vi "De-Classify Error Call Chain.vi"(8 "Classified Error":errorcluster) -> (0 "De-Classified Error":errorcluster, 2 "Classification Detected":bool, 3 "Error Classification":string)   [LabVIEW 2019, in "Logger.Error.lvclass"]
doc: "This VI returns and removes \"classification\" information that was previously attached to an error using the Classify Error VI or the Specific Error Handler. This VI is typically called as part of a Central Error Handler. This VI modifies the source string of the error to remove the classification."
uses:
  Logger.Error.lvclass
  <vilib>/regexp/Match Regular Expression.xnode
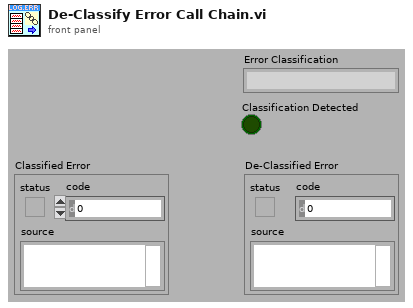
[diagram p1: front panel]
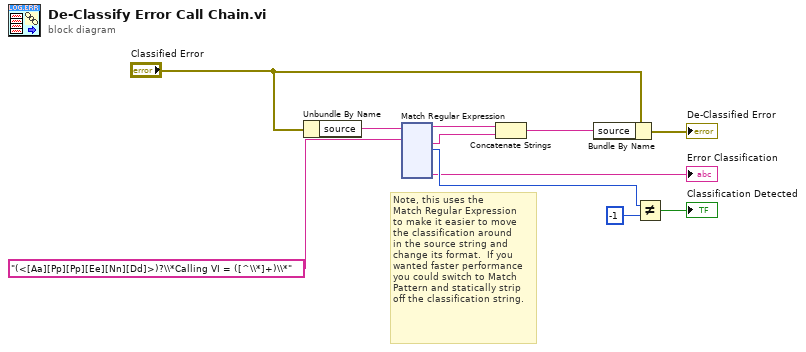
[diagram p0: block diagram]
diagram:
  # "Note, this uses the\nMatch Regular Expression\nto make it easier to move\nthe classification around\nin the source string and\nchange its format.  If you\nwanted faster performance\nyou could switch to Match\nPattern and statically strip\noff the classification string."
  n1 = Unbundle By Name("Classified Error") -> ("source"=w6:string)
  n2 = xnode "Match Regular Expression"("input string"=w6, "regular expression"="(<[Aa][Pp][Pp][Ee][Nn][Dd]>)?\\*Calling VI = ([^\\*]+)\\*" ("regular expression (\"\")")) -> ("before match"=w4:string, "after match"=w3:string, "offset past match"=w2:i32, "submatch 2"=→"Error Classification":string)  [unwired: 2 in, 5 out]
  n3 = Concatenate Strings(w4, w3) -> (w8:string)
  n4 = Bundle By Name(cluster="Classified Error", "source"=w8) -> (→"De-Classified Error":errorcluster)
  n5 = Not Equal?(x=w2, y=-1) -> (x != y?=→"Classification Detected":bool)
